vi "Message.vi"() -> ()   [LabVIEW 2017, in "Assertions.Tests.lvlib" / "Assert Error.lvlib"]
uses:
  Assert Error.lvlib
  src/Transparent Assertions/Assertions/Assertions.lvlib
panel:
  out "error out":errorcluster
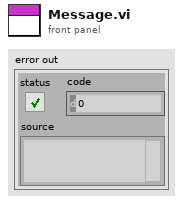
[diagram p1: front panel]
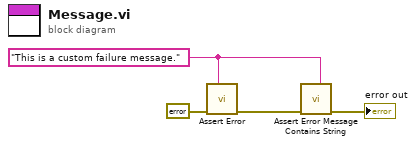
[diagram p0: block diagram]
diagram:
  w1 = "This is a custom failure message." ("Message (\"\")")
  n1 = call "Assert Error.vi"("Message (\"\")"=w1, "error in (no error)"=errorcluster {"status"=FALSE, "code"=0, "source"=""}) -> ("error out"=w3:errorcluster)  [unwired: 9 in]
  n2 = call "Assert Error Message Contains String.vi"("Expected"=w1, "error in (no error)"=w3) -> ("error out"=→"error out":errorcluster)  [unwired: 9 in]
